vi "Format Date.vi"(0 "Time Stamp In":timestamp) -> (4 "Formatted DateTime Out":string, 6 "Filename Date Time Out":string, 8 "Filename Date Out":string, 10 "Formatted Date Out":string, 15 "Formatted Time Out":string)   [LabVIEW 2024, in "LVarex.lvlib"]
uses:
  LVarex.lvlib
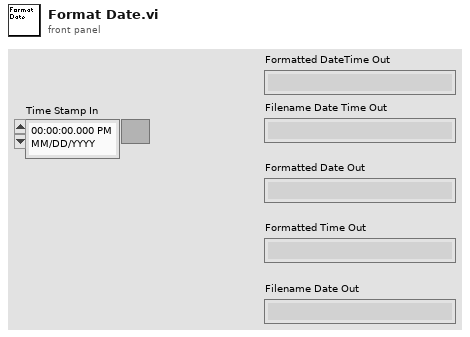
[diagram p1: front panel]
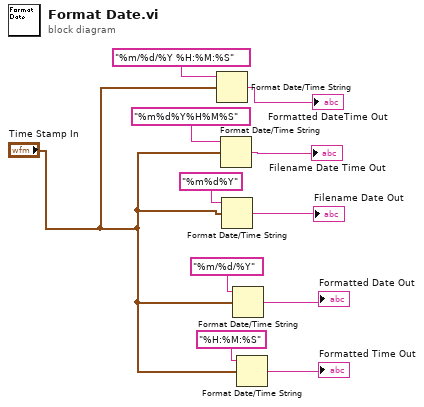
[diagram p0: block diagram]
diagram:
  n1 = Format Date/Time String(time format string (%c)="%m/%d/%Y %H:%M:%S", seconds (now)="Time Stamp In") -> (date/time string=→"Formatted DateTime Out":string)  [unwired: 1 in]
  n2 = Format Date/Time String(time format string (%c)="%m%d%Y%H%M%S", seconds (now)="Time Stamp In") -> (date/time string=→"Filename Date Time Out":string)  [unwired: 1 in]
  n3 = Format Date/Time String(time format string (%c)="%m%d%Y", seconds (now)="Time Stamp In") -> (date/time string=→"Filename Date Out":string)  [unwired: 1 in]
  n4 = Format Date/Time String(time format string (%c)="%m/%d/%Y", seconds (now)="Time Stamp In") -> (date/time string=→"Formatted Date Out":string)  [unwired: 1 in]
  n5 = Format Date/Time String(time format string (%c)="%H:%M:%S", seconds (now)="Time Stamp In") -> (date/time string=→"Formatted Time Out":string)  [unwired: 1 in]
